vi "Remove Comments from XML.vi"(11 "XML String in":string) -> (3 "XML String out":string)   [LabVIEW 2020, in "NI_VIAn_XML Parsing.lvlib"]
uses:
  <vilib>/addons/analyzer/XML Parsing/NI_VIAn_XML Parsing.lvlib
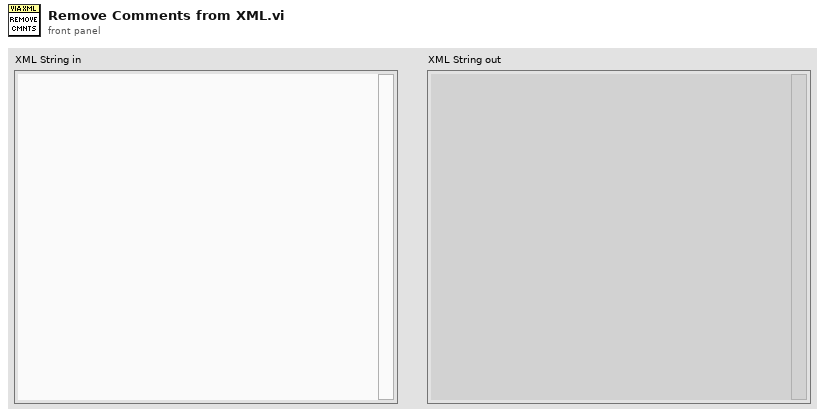
[diagram p1: front panel]
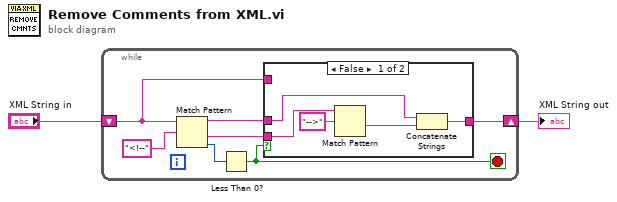
[diagram p0: block diagram]
diagram:
  n1 = while {
    shift-right: [w6] -> w1
    shift-left: "XML String in" -> [w7]
    stop <- w8 stop-if-true
    n2 = Match Pattern(string=w7, regular expression="<!--") -> (before substring=w4:string, after substring=w3:string, offset past match=w9:i32)  [unwired: 1 in, 1 out]
    n3 = Less Than 0?(x=w9) -> (x < 0?=w8:bool)
    n4 = case shown="False" w8 {
      tunnel: w7 -> [_ w15]
      tunnel: [w11 w15] -> w6
      tunnel: w4 -> [w12 _]
      tunnel: w3 -> [w14 _]
      frame False {
        n5 = Match Pattern(string=w14, regular expression="-->") -> (after substring=w10:string)  [unwired: 1 in, 3 out]
        n6 = Concatenate Strings(w12, w10) -> (w11:string)
      }
      frame True {
      }
    }
  }
  "XML String out" <- w1
